vi "Read_Ch_data_file.vi"(5 "Present Channels only":bool=TRUE, 6 "Start of read offset (chars.: 0)":i32, 7 "Present Channels":string[](array[string]), 8 "Output":enum16{"All Ch data", "The last few rows"}(ring), 9 "Filename":path) -> (0 "Merged?":bool, 1 "Channel Values":string[][](array[string]), 2 "Merged Channels":string[](array[string]), 3 "exists?":bool=TRUE, 4 "Offset from File End":i32)   [LabVIEW 2010]
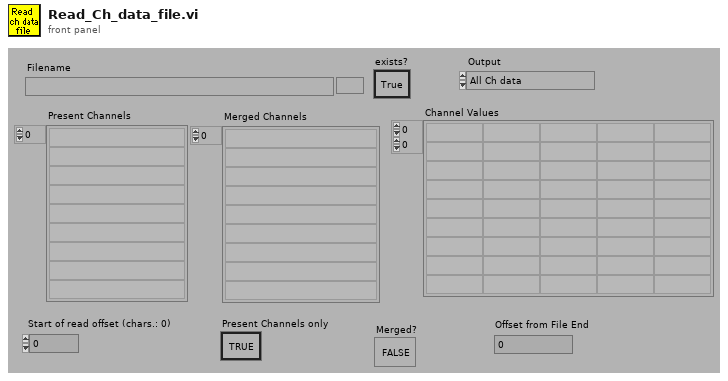
[diagram p1: front panel]
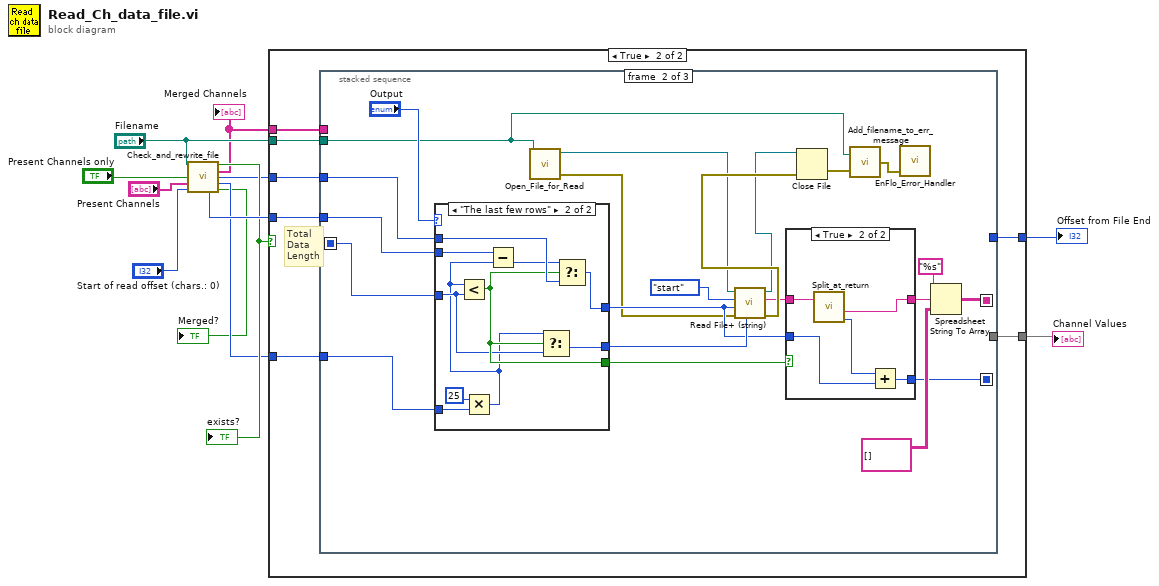
[diagram p0: block diagram]
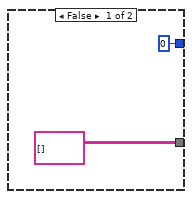
[diagram p2: hidden frame]
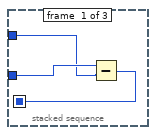
[diagram p3: hidden frame]
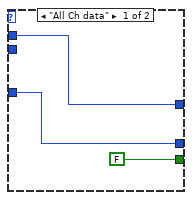
[diagram p5: hidden frame]
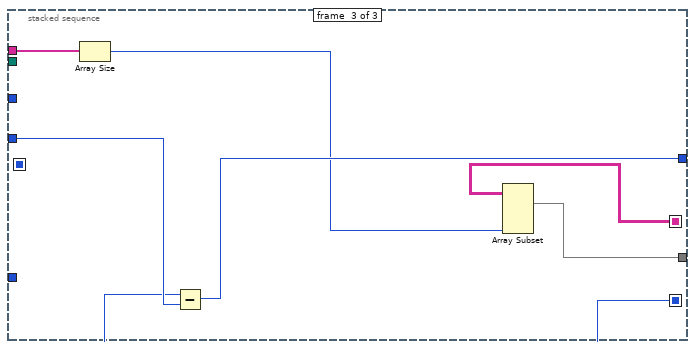
[diagram p6: hidden frame]
diagram:
  n1 = call "Check_and_rewrite_file.vi"("Filename"="Filename", "Present Channels only"="Present Channels only", "Present Channels"="Present Channels", "Start of read offset (chars.: 0)"="Start of read offset (chars.: 0)") -> ("exists?"=w6:bool, "Merged Channels"=w1:string[], "Start of data (bytes)"=w4:i32, "No of bytes/row (approx)"=w5:i32, "Current file size (bytes)"=w7:i32, "Merged?"=→"Merged?":bool)  [unwired: 6 out]
  "exists?" <- w6
  "Merged Channels" <- w1
  n2 = case shown="True" w6 {
    tunnel: [string[][] [] ("Channel Values") w20] -> w12
    tunnel: "Filename" -> [_ w21]
    tunnel: w7 -> [_ w19]
    tunnel: [0 w18] -> w11
    tunnel: w5 -> [_ w17]
    tunnel: w4 -> [_ w16]
    tunnel: w1 -> [_ w15]
    frame False {
    }
    frame True {
      # "Total\nData\nLength"
      n3 = stacked-sequence {
        seq-local: [_ w40 _] -> [_ _ w71]
        seq-local: [w23 _ _] -> [_ w37 _]
        seq-local: [_ w29 _] -> [_ _ w67]
        tunnel: w21 -> [_ w25 _]
        tunnel: [_ _ w68] -> w20
        tunnel: w19 -> [w24 w38 w72]
        tunnel: [_ _ w73] -> w18
        tunnel: w17 -> [_ w32 _]
        tunnel: w16 -> [w22 w31 _]
        tunnel: w15 -> [_ _ w70]
        frame #0 {
          n4 = Subtract(x=w24, y=w22) -> (x-y=w23:i32)
        }
        frame #1 {
          n5 = case shown="\"The last few rows\"" "Output" {
            tunnel: w31 -> [w56 w64]
            tunnel: [w56 w60] -> w41
            tunnel: [w54 w61] -> w46
            tunnel: w38 -> [_ w59]
            tunnel: [FALSE w63] -> w42
            tunnel: w32 -> [_ w65]
            tunnel: w37 -> [w54 w62]
            frame "All Ch data" {
            }
            frame "The last few rows" {
              n6 = Multiply(x=25 ("offset"), y=w65) -> (x*y=w58:i32)
              n7 = Less?(x=w58, y=w62) -> (x < y?=w63:bool)
              n8 = Subtract(x=w59, y=w58) -> (x-y=w57:i32)
              n9 = Select(t=w58, s=w63, f=w62) -> (s? t:f=w61:i32)
              n10 = Select(t=w57, s=w63, f=w64) -> (s? t:f=w60:i32)
            }
          }
          n11 = call "Open_File_for_Read.vi"("file path"=w25) -> ("error out"=w36:errorcluster, "refnum"=w28:refnum<file>)  [unwired: 1 in, 8 out]
          n12 = call <vilib>:"Read File+ (string).vi"("count"=w46, "error in (no error)"=w36, "pos offset (bytes:0)"=w41, "pos mode (rel. to current:2)"=enum16{"start", "end", "current"}."start" ("pos mode (0:2)"), "refnum"=w28) -> ("error out"=w44:errorcluster, "string"=w30:string, "dup refnum"=w39:refnum<file>)  [unwired: 4 out]
          n13 = case shown="True" w42 {
            tunnel: w30 -> [w48 w50]
            tunnel: [w48 w51] -> w34
            tunnel: w41 -> [w47 w53]
            tunnel: [w47 w52] -> w40
            frame False {
            }
            frame True {
              n14 = call "Split_at_return.vi"("String"=w50) -> ("after substring"=w51:string, "offset past match"=w49:i32)  [unwired: 1 in, 2 out]
              n15 = Add(x=w49, y=w53) -> (x+y=w52:i32)
            }
          }
          n16 = Close File(refnum=w39, error in=w44) -> (error out=w27:errorcluster)  [unwired: 1 out]
          n17 = call "Add_filename_to_err_message.vi"("error in (no error)"=w27, "Path"=w25) -> ("error out"=w26:errorcluster)
          n18 = call "EnFlo_Error_Handler.vi"("error in (no error)"=w26) -> ()  [unwired: 2 in, 3 out]
          n19 = Spreadsheet String To Array(format string="%s", spreadsheet string=w34, array type (2D Dbl)=string[][] [] ("Channel Values")) -> (array=w29:string[][])  [unwired: 1 out]
        }
        frame #2 {
          n20 = Array Size(array=w70) -> (size(s)=w69:i32)
          n21 = Subtract(x=w71, y=w72) -> (x-y=w73:i32)
          n22 = Array Subset(array=w67, length (col)=w69) -> (w68:string[][])  [unwired: 3 in]
        }
      }
    }
  }
  "Channel Values" <- w12
  "Offset from File End" <- w11
